vi "Read and Error Query.vi"(8 "error in (no error)":errorcluster, 10 "Bytes To Read (0)":u32, 11 "VISA resource name":refnum<visa-resource-name>) -> (0 "error out":errorcluster, 3 "VISA resource name out":refnum<visa-resource-name>)   [LabVIEW 2012, in "MicroStrain 3DM-GXx.lvlib"]
doc: "Reads the instrument response and performs a checksum to notify user of any instrument errors."
uses:
  <instrlib>/MicroStrain 3DM-GXx/MicroStrain 3DM-GXx.lvlib
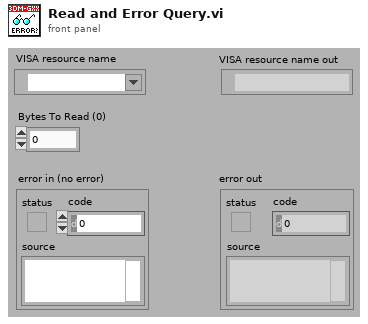
[diagram p1: front panel]
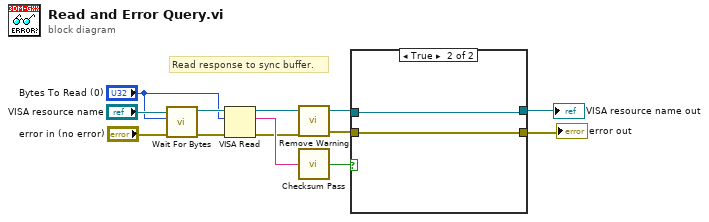
[diagram p0: block diagram]
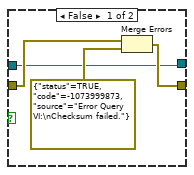
[diagram p2: hidden frame]
diagram:
  # "Read response to sync buffer."
  n1 = call <instrlib>:"Wait For Bytes.vi"("error in (no error)"="error in (no error)", "Bytes To Read (0)"="Bytes To Read (0)", "VISA resource name"="VISA resource name") -> ("error out"=w12:errorcluster, "VISA resource name out"=w13:refnum<visa-resource-name>)  [unwired: 7 in]
  n2 = VISA Read(VISA resource name=w13, byte count="Bytes To Read (0)", error in (no error)=w12) -> (VISA resource name out=w10:refnum<visa-resource-name>, read buffer=w11:string, error out=w9:errorcluster)  [unwired: 1 out]
  n3 = call <instrlib>:"Remove Warning.vi"("error in (no error)"=w9, "VISA resource name"=w10) -> ("error out"=w7:errorcluster, "VISA resource name out"=w6:refnum<visa-resource-name>)  [unwired: 2 in]
  n4 = call <instrlib>:"Checksum Pass.vi"("Message In"=w11) -> ("Checksum Pass"=w8:bool)  [unwired: 4 in]
  n5 = case shown="True" w8 {
    tunnel: w7 -> [w17 w19]
    tunnel: [w16 w19] -> w1
    tunnel: [w14 w18] -> w4
    tunnel: w6 -> [w14 w18]
    frame False {
      n6 = Merge Errors(w17, errorcluster {"status"=TRUE, "code"=-1073999873, "source"="Error Query VI:\nChecksum failed."} ("error in 2 (no error)")) -> (w16:errorcluster)
    }
    frame True {
    }
  }
  "error out" <- w1
  "VISA resource name out" <- w4
